vi "UnboxDouble.vi"(10 "Double in":refnum<class "Double.lvclass">) -> (2 "Numeric":dbl)   [LabVIEW 2013, in "LapDog.Collections.v1.Common.lvlib" / "Double.lvclass"]
uses:
  Double.lvclass
  Double.lvclass/Double.ctl
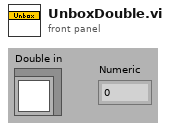
[diagram p1: front panel]
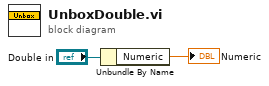
[diagram p0: block diagram]
diagram:
  n1 = Unbundle By Name("Double in") -> ("Numeric"=→"Numeric":dbl)
